vi "set mapping type array by channel.vi"(7 "owner ID":string, 8 "error in":errorcluster, 9 "Mapping":T1, 10 "channel":refnum<class "TBM channel.lvclass">, 11 "engine configuration in":refnum<class "engine configuration.lvclass">) -> (0 "error out":errorcluster, 3 "engine configuration out":refnum<class "engine configuration.lvclass">)   [LabVIEW 2013, in "engine configuration.lvclass"]
uses:
  engine configuration.lvclass
  <vilib>/NI/Tag Bus Module Framework/channel/TBM channel.lvclass
  <vilib>/NI/Tag Bus/table/mapping specification.ctl
  <vilib>/NI/Tag Bus/tag/Data Type.ctl
  <vilib>/NI/Tag Bus/table/mapping.ctl
  engine configuration.lvclass/engine configuration.ctl
  <vilib>/NI/Tag Bus/tag/tag descriptor.lvclass/tag descriptor.ctl
  <vilib>/NI/Tag Bus/tag/read data type.vi
  <vilib>/NI/Tag Bus/tag/read tag name.vi
  <vilib>/NI/Tag Bus Module Framework/root configuration/TBM configuration.lvclass
  <vilib>/NI/Tag Bus/tag/tag descriptor.lvclass
  <vilib>/NI/Tag Bus/table/data table.lvlib
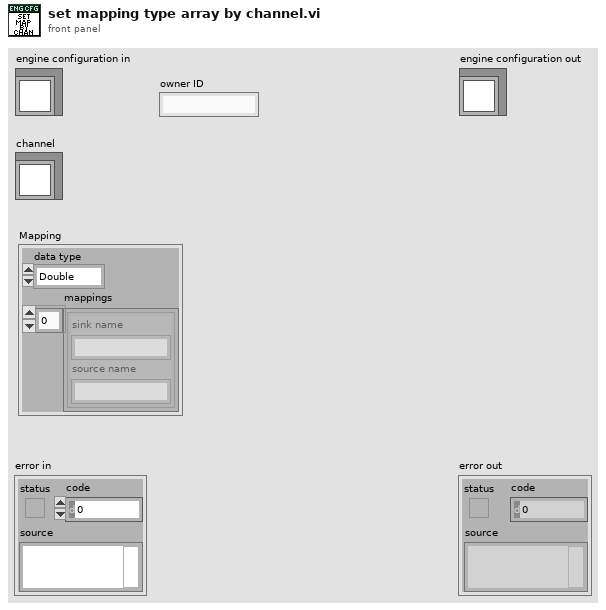
[diagram p1: front panel]
types:
  T1 = typedef "tag bus.lvlib/data table.lvlib/mapping specification.ctl" = cluster{"data type":T2, "mappings":T3[]}
  T2 = typedef "tag bus.lvlib/tag descriptor.lvclass/Data Type.ctl" = enum16{"Double", "Single", "I64", "I32", "I16", "I8", "U64", "U32", "U16", "U8", "Boolean", "String", "Array of Double", "Array of Single", "Array of I64", "Array of I32", "Array of I16", "Array of I8", "Array of U64", "Array of U32", "Array of U16", "Array of U8", "Array of Boolean", "Array of String"}
  T3 = typedef "tag bus.lvlib/data table.lvlib/mapping.ctl" = cluster{"sink name":string, "source name":string}
  T4 = typedef "engine configuration.lvclass/Module Mappings.ctl" = cluster{"Owning ID":string, "Input Mappings":T1[], "Process Parameter Mappings":T1[], "Process Results Mappings":T1[], "Output Mappings":T1[]}
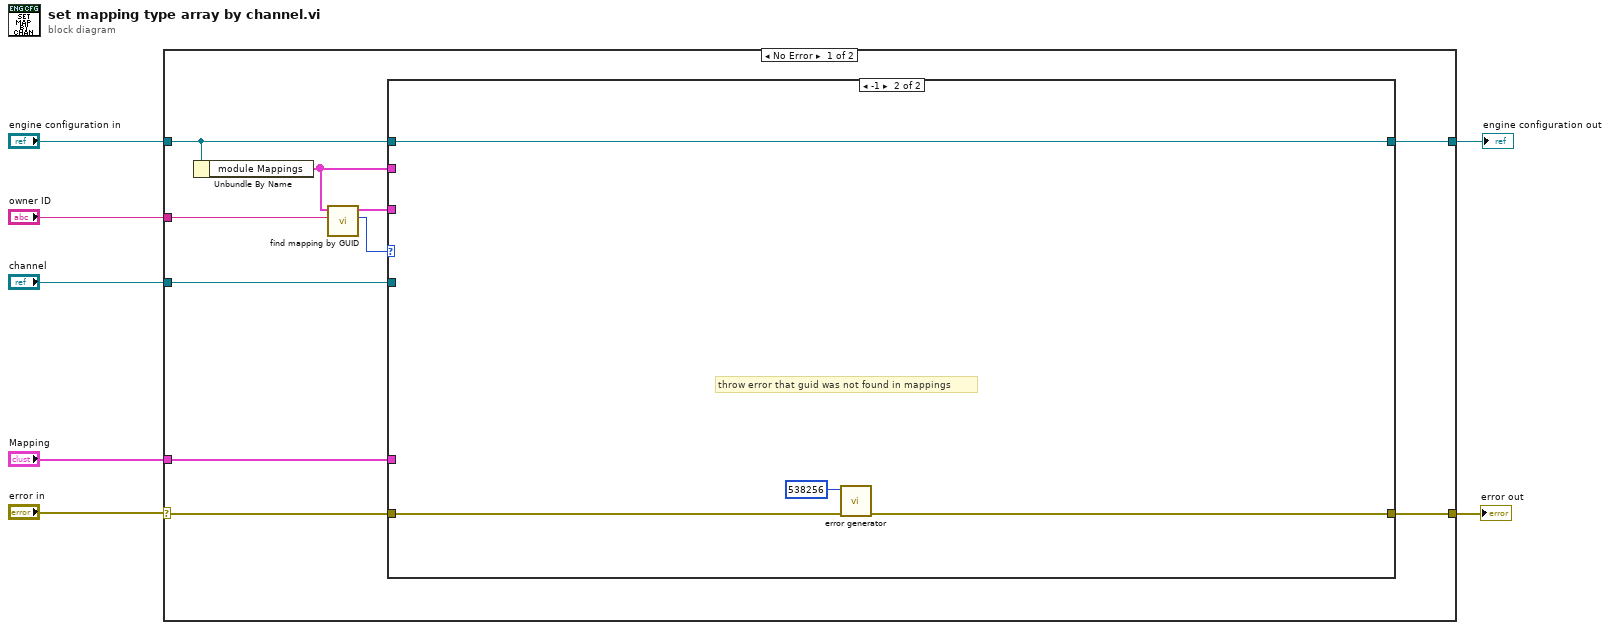
[diagram p0: block diagram]
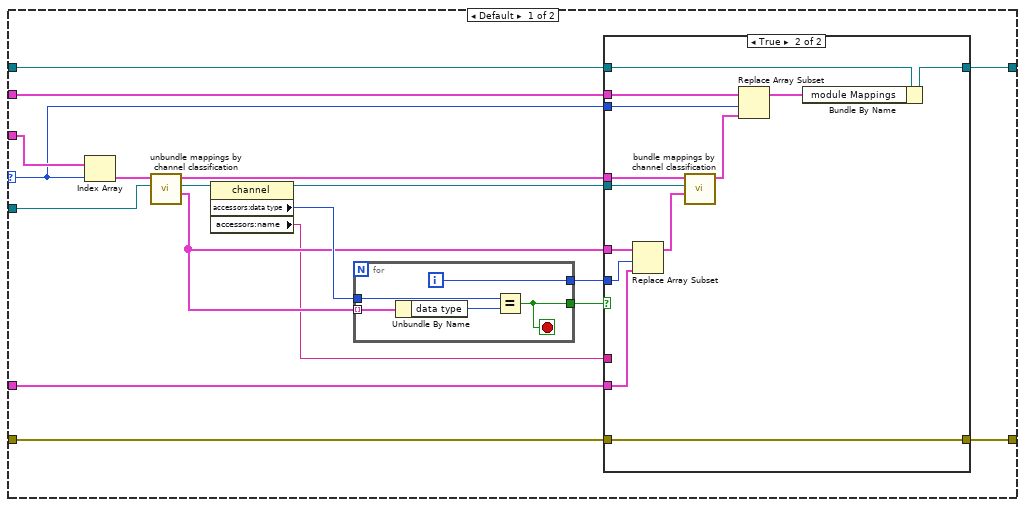
[diagram p2: hidden frame]
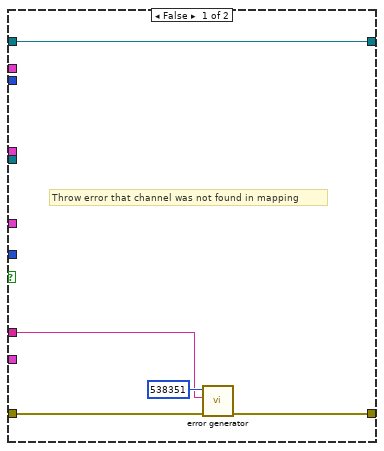
[diagram p3: hidden frame]
diagram:
  n1 = case shown="No Error" "error in" {
    selector: "error in" -> [w9 w64]
    tunnel: [w8 w64] -> w2
    tunnel: [w10 w63] -> w1
    tunnel: "engine configuration in" -> [w13 w63]
    tunnel: "owner ID" -> [w17 _]
    tunnel: "channel" -> [w14 _]
    tunnel: "Mapping" -> [w11 _]
    frame No Error {
      n2 = Unbundle By Name(w13) -> ("module Mappings"=w12:T4[])
      n3 = call "find mapping by GUID.vi"("owner ID"=w17, "module Mappings"=w12) -> ("index"=w16:i32, "module Mappings out"=w15:T4[])  [unwired: 8 in]
      n4 = case shown="-1" w16 {
        selector: w16 -> [w26 _]
        tunnel: w15 -> [w35 _]
        tunnel: w14 -> [w33 _]
        tunnel: w13 -> [w28 w62]
        tunnel: w12 -> [w27 _]
        tunnel: w11 -> [w24 _]
        tunnel: [w21 w62] -> w10
        tunnel: w9 -> [w20 w60]
        tunnel: [w19 w59] -> w8
        frame Default {
          n5 = Index Array(array=w35, index=w26) -> (element=w34:T4)
          n6 = call "unbundle mappings by channel classification.vi"("channel"=w33, "Mappings"=w34) -> ("Mappings For One Method"=w22:T1[], "channel out"=w32:refnum<class "TBM channel.lvclass">, "Mappings out"=w23:T4)  [unwired: 7 in]
          n7 = property class="channel"(reference=w32) -> (reference out=w25:refnum<class "TBM channel.lvclass">, "accessors:data type"=w31:T2, "accessors:name"=w18:string)  [unwired: 1 in, 1 out]
          n8 = for {
            tunnel: w22 -> [w54] mode=indexing
            tunnel: w31 -> [w57]
            tunnel: [w56] -> w30
            tunnel: [w55] -> w29
            i -> [w55]
            stop <- w56 stop-if-true
            n9 = Unbundle By Name(w54) -> ("data type"=w58:T2)
            n10 = Equal?(x=w57, y=w58) -> (x = y?=w56:bool)
          }
          n11 = case shown="True" w30 {
            tunnel: w29 -> [_ w52]
            tunnel: w28 -> [w40 w44]
            tunnel: w27 -> [_ w47]
            tunnel: w26 -> [_ w46]
            tunnel: w25 -> [_ w49]
            tunnel: w24 -> [_ w51]
            tunnel: w23 -> [_ w50]
            tunnel: w22 -> [_ w53]
            tunnel: [w40 w42] -> w21
            tunnel: w20 -> [w38 w41]
            tunnel: [w36 w41] -> w19
            tunnel: w18 -> [w37 _]
            frame False {
              # "Throw error that channel was not found in mapping"
              n12 = call <vilib>:"error generator.vi"("error in"=w38, "append error message"=w37, "error code (0)"=538351) -> ("error out"=w36:errorcluster)  [unwired: 8 in]
            }
            frame True {
              n13 = Replace Array Subset(array=w53, new element=w51, index=w52) -> (w48:T1[])
              n14 = call "bundle mappings by channel classification.vi"("Mappings For One Method"=w48, "channel"=w49, "Mappings"=w50) -> ("Mappings out"=w45:T4)  [unwired: 7 in, 1 out]
              n15 = Replace Array Subset(array=w47, new element=w45, index=w46) -> (w43:T4[])
              n16 = Bundle By Name(cluster=w44, "module Mappings"=w43) -> (w42:refnum<class "engine configuration.lvclass">)
            }
          }
        }
        frame -1 {
          # "throw error that guid was not found in mappings"
          n17 = call <vilib>:"error generator.vi"("error in"=w60, "error code (0)"=538256) -> ("error out"=w59:errorcluster)  [unwired: 9 in]
        }
      }
    }
    frame Error {
    }
  }
  "error out" <- w2
  "engine configuration out" <- w1
